vi "SMC Global.vi"() -> ()   [LabVIEW 2009]
panel:
  in  "IPS Device":string
  in  "Witness Device":string
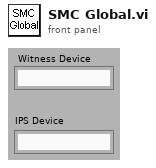
[diagram p1: front panel]
diagram:
